vi "TCP_StatusCheck.vi"(8 "error in (no error)":errorcluster, 10 "Clients":refnum<k5>[](array[refnum]), 11 "listener ID in":refnum<k5>) -> (0 "no error":errorcluster, 2 "Clients":refnum<k5>[](array[refnum]), 3 "SenData":bool)   [LabVIEW 2020, in "TCP_Server.lvlib"]
uses:
  TCP_Server.lvlib
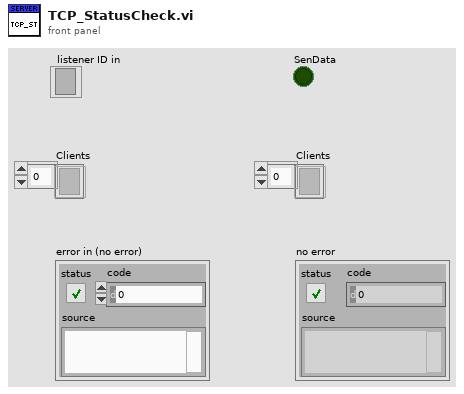
[diagram p1: front panel]
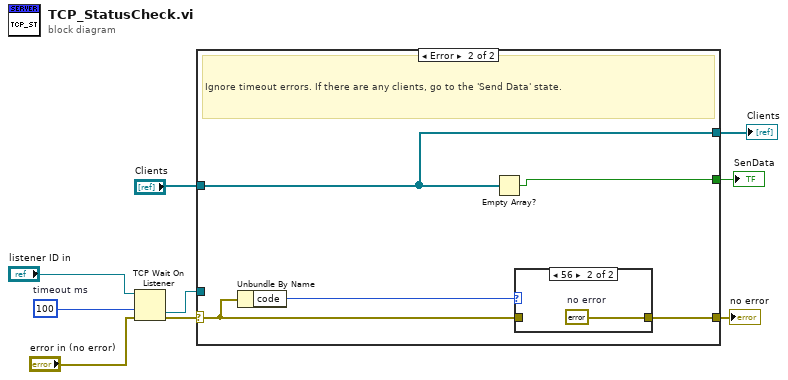
[diagram p0: block diagram]
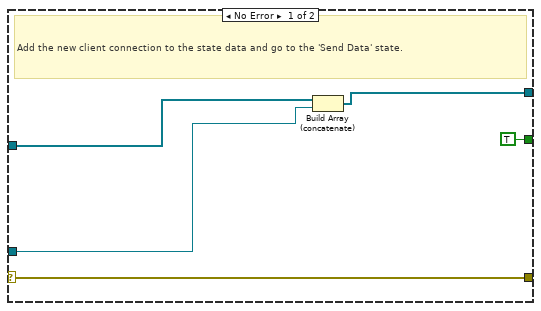
[diagram p2: hidden frame]
diagram:
  w9 = 100  # timeout ms
  n1 = TCP Wait On Listener(8:"error in (no error)", 9:w9, 11:"listener ID in") -> (0:w8:errorcluster, 4:w7:refnum<k5>)  [unwired: 4 out]
  n2 = case shown="Error" w8 {
    selector: w8 -> [w13 w19]
    tunnel: w7 -> [w14 _]
    tunnel: [w13 w17] -> w2
    tunnel: "Clients" -> [w11 w15]
    tunnel: [TRUE ("empty?") w16] -> w4
    tunnel: [w12 w15] -> w3
    frame No Error {
      # "Add the new client connection to the state data and go to the 'Send Data' state."
      n3 = Build Array (concatenate)(w11, w14) -> (w12:refnum<k5>[])
    }
    frame Error {
      # "Ignore timeout errors. If there are any clients, go to the 'Send Data' state."
      n4 = Unbundle By Name(w19) -> ("code"=w18:i32)
      n5 = Empty Array?(array=w15) -> (empty?=w16:bool)
      n6 = case shown="56" w18 {
        tunnel: w19 -> [w20 _]
        tunnel: [w20 w21] -> w17
        frame Default {
        }
        frame 56 {
          w21 = errorcluster {"status"=FALSE, "code"=0, "source"=""}  # no error
        }
      }
    }
  }
  "SenData" <- w4
  "Clients" <- w3
  "no error" <- w2
